vi "Get Project Data From File.vi"(8 "error in (no error)":errorcluster, 11 "TS UI Data in":T1) -> (0 "error out":errorcluster, 3 "TS UI Data out":T1)   [LabVIEW 2015]
uses:
  <vilib>/Utility/config.llb/NI_LVConfig.lvlib
  <vilib>/Utility/config.llb/Read Key (String).vi
  Type defs/TS UI Data.ctl
  Type defs/Nest cluster.ctl
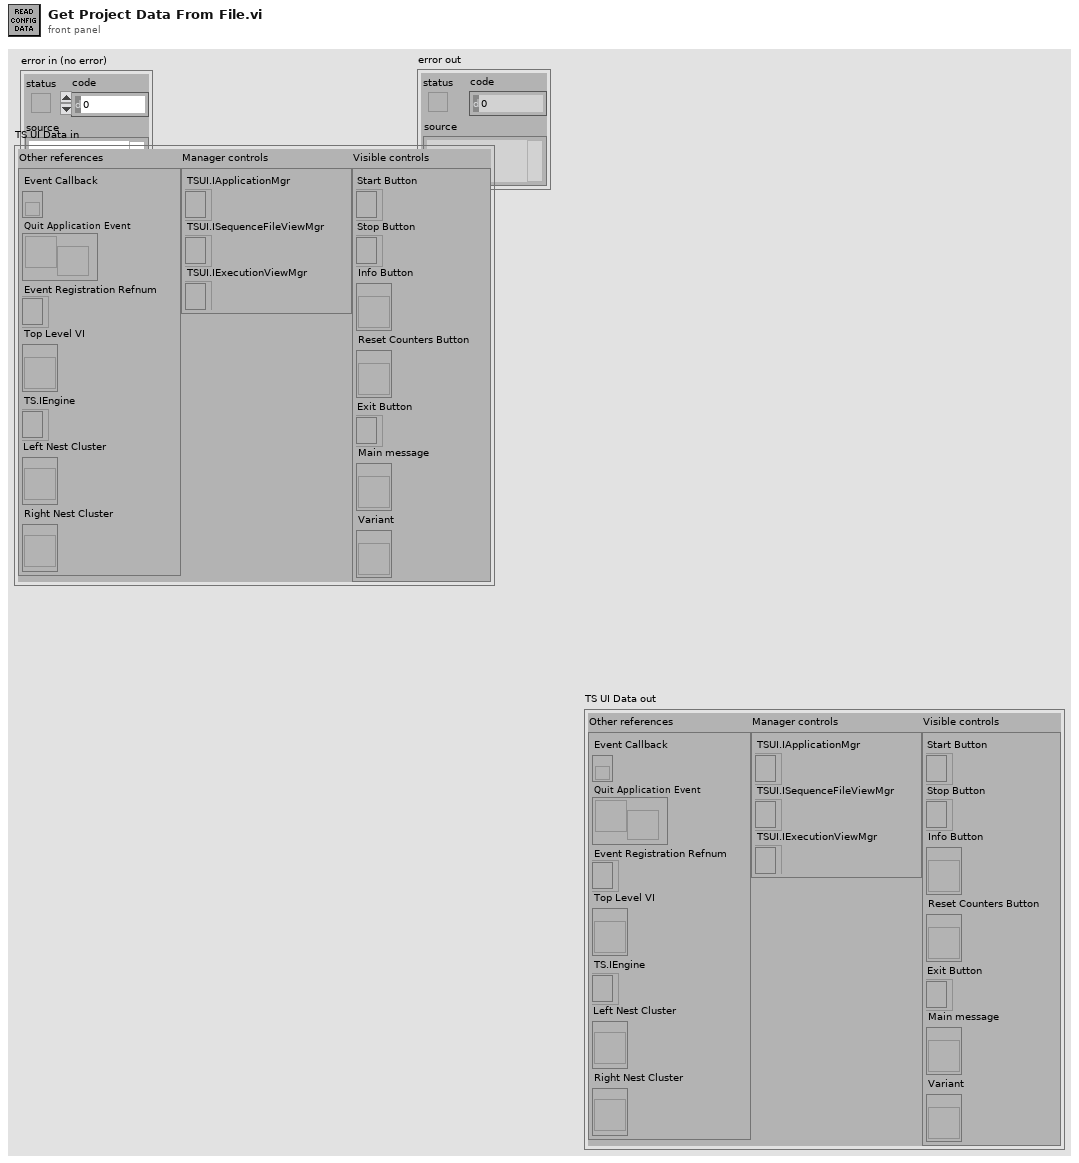
[diagram p1: front panel]
types:
  T1 = typedef "TS UI Data.ctl" = cluster{"Other references":cluster{"Event Callback":refnum<k27>, "Quit Application Event":refnum<user-event>, "event registration refnum":refnum<event-registration>, "Top Level VI":refnum<vi>, "TS.IEngine":refnum<k7>, "Left Nest Cluster":refnum<vi>, "Right Nest Cluster":refnum<vi>}, "Manager controls":cluster{"TSUI.IApplicationMgr":refnum<k7>, "TSUI.ISequenceFileViewMgr":refnum<k7>, "TSUI.IExecutionViewMgr":refnum<k7>}, "Visible controls":cluster{"Start Button":refnum<k7>, "Stop Button":refnum<k7>, "Info Button":refnum<vi>, "Reset Counters Button":refnum<vi>, "Exit Button":refnum<k7>, "Main message":refnum<vi>, "Variant":refnum<vi>}}
  T2 = typedef "NI_LVConfig.lvlib/Config Data RefNum.ctl" = refnum<k1>
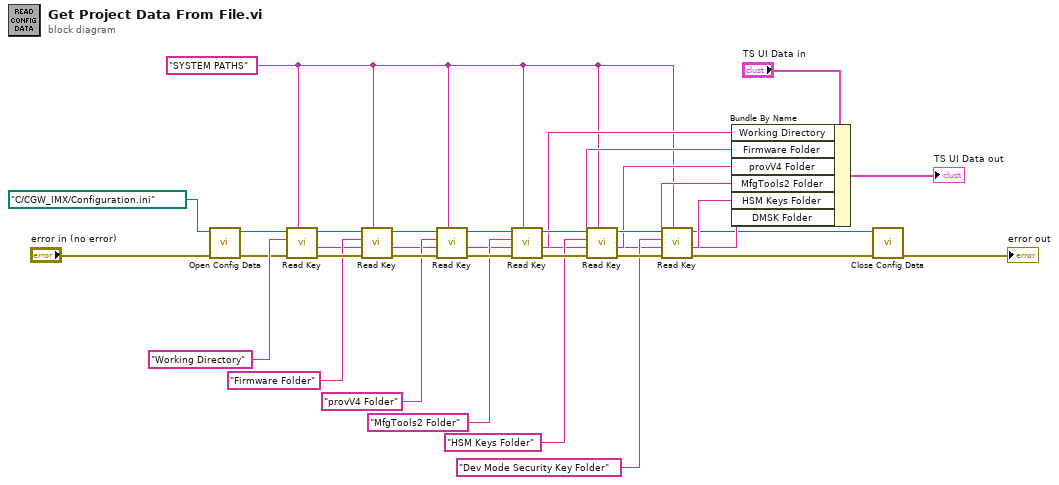
[diagram p0: block diagram]
diagram:
  w4 = "SYSTEM PATHS"
  n1 = call <vilib>:"Open Config Data.vi"("error in (no error)"="error in (no error)", "configuration file path"=path "C:/CGW_IMX/Configuration.ini") -> ("error out"=w9:errorcluster, "refnum"=w10:T2)  [unwired: 7 in, 1 out]
  n2 = call-poly <vilib>:"Read Key.vi"("section"=w4, "error in (no error)"=w9, "key"="Working Directory", "refnum"=w10) -> ("error out"=w30:errorcluster, "value"=w16:string, "refnum out"=w31:T2)  [unwired: 4 in, 1 out]
  n3 = call-poly <vilib>:"Read Key.vi"("section"=w4, "error in (no error)"=w30, "key"="Firmware Folder", "refnum"=w31) -> ("error out"=w29:errorcluster, "value"=w15:string, "refnum out"=w25:T2)  [unwired: 4 in, 1 out]
  n4 = call-poly <vilib>:"Read Key.vi"("section"=w4, "error in (no error)"=w29, "key"="provV4 Folder", "refnum"=w25) -> ("error out"=w28:errorcluster, "value"=w14:string, "refnum out"=w24:T2)  [unwired: 4 in, 1 out]
  n5 = call-poly <vilib>:"Read Key.vi"("section"=w4, "error in (no error)"=w28, "key"="MfgTools2 Folder", "refnum"=w24) -> ("error out"=w27:errorcluster, "value"=w13:string, "refnum out"=w23:T2)  [unwired: 4 in, 1 out]
  n6 = call-poly <vilib>:"Read Key.vi"("section"=w4, "error in (no error)"=w27, "key"="HSM Keys Folder", "refnum"=w23) -> ("error out"=w26:errorcluster, "value"=w12:string, "refnum out"=w22:T2)  [unwired: 4 in, 1 out]
  n7 = call-poly <vilib>:"Read Key.vi"("section"=w4, "error in (no error)"=w26, "key"="Dev Mode Security Key Folder", "refnum"=w22) -> ("error out"=w6:errorcluster, "value"=w11:string, "refnum out"=w7:T2)  [unwired: 4 in, 1 out]
  n8 = Bundle By Name(cluster="TS UI Data in", "Working Directory"=w16, "Firmware Folder"=w15, "provV4 Folder"=w14, "MfgTools2 Folder"=w13, "HSM Keys Folder"=w12, "DMSK Folder"=w11) -> (→"TS UI Data out":T1)
  n9 = call <vilib>:"Close Config Data.vi"("error in (no error)"=w6, "refnum"=w7) -> ("error out"=→"error out":errorcluster)  [unwired: 8 in, 1 out]
